vi "[Template] - State Machine Module.vi"() -> ()   [LabVIEW 2015]
uses:
  TypeDefs/ENUM_State Template.ctl
  TypeDefs/ENUM_Request Template.ctl
  Utility/Universal Utility/FP/FPClass/(FP)/DecFrame_FP/DecFrame_FP.lvclass
  <vilib>/Utility/error.llb/DialogType.ctl
  Utility/Universal Utility/TypeDefs_Utility/ENUM RB_Pos_Quadrant Position.ctl
  <vilib>/Utility/error.llb/Trim Whitespace.vi
panel:
  in  "stop":bool
  out "Version":string
  out "Action":string
  out "Next Request":T1 caption="Request ENUM (REPLACE)"
  out "State":T2=enum."Idle" caption="State ENUM (REPLACE)"
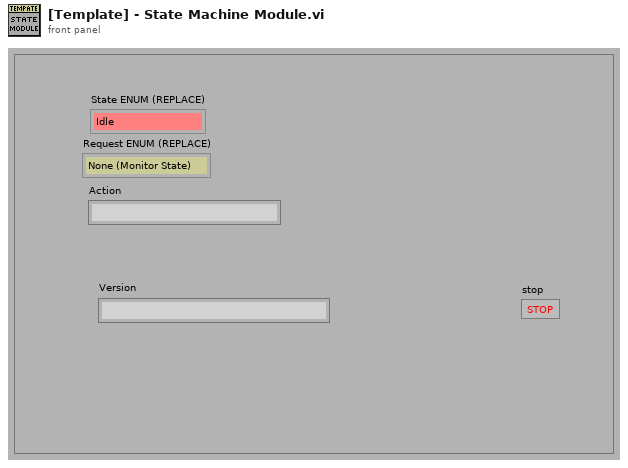
[diagram p1: front panel]
types:
  T1 = typedef "ENUM_Request Template.ctl" = enum16{"None (Monitor State)", "Request 1", "Stop Program", "SetFP Request"}
  T2 = typedef "ENUM_State Template.ctl" = enum16{"<Startup>", "Idle", "STATE 1", "<Shutdown>"}
  T3 = enum32{"invalid app kind", "Development System", "Run Time System", "Student Edition", "Embedded LabVIEW", "Evaluation", "Custom"}
  T4 = cluster{"App Kind":enum32{"invalid app kind", "Development System", "Run Time System", "Student Edition", "Embedded LabVIEW", "Evaluation", "Custom"}, "This VI":refnum<vi>, "Timeout":i32, "State":T2, "Request Q":refnum<queue>, "FP Data":refnum<class "DecFrame_FP.lvclass">}
  T5 = typedef "ENUM RB_Pos_Quadrant Position.ctl" = enum32{"LFT-TOP", "MID-TOP", "RGT-TOP", "LFT-CTR", "MID-CTR", "RGT-CTR", "LFT-BOT", "MID-BOT", "RGT-BOT"}
  T6 = enum32{"Invalid", "Standard", "Closed", "Hidden", "Minimized", "Maximized"}
  T7 = typedef "DialogType.ctl" = u16
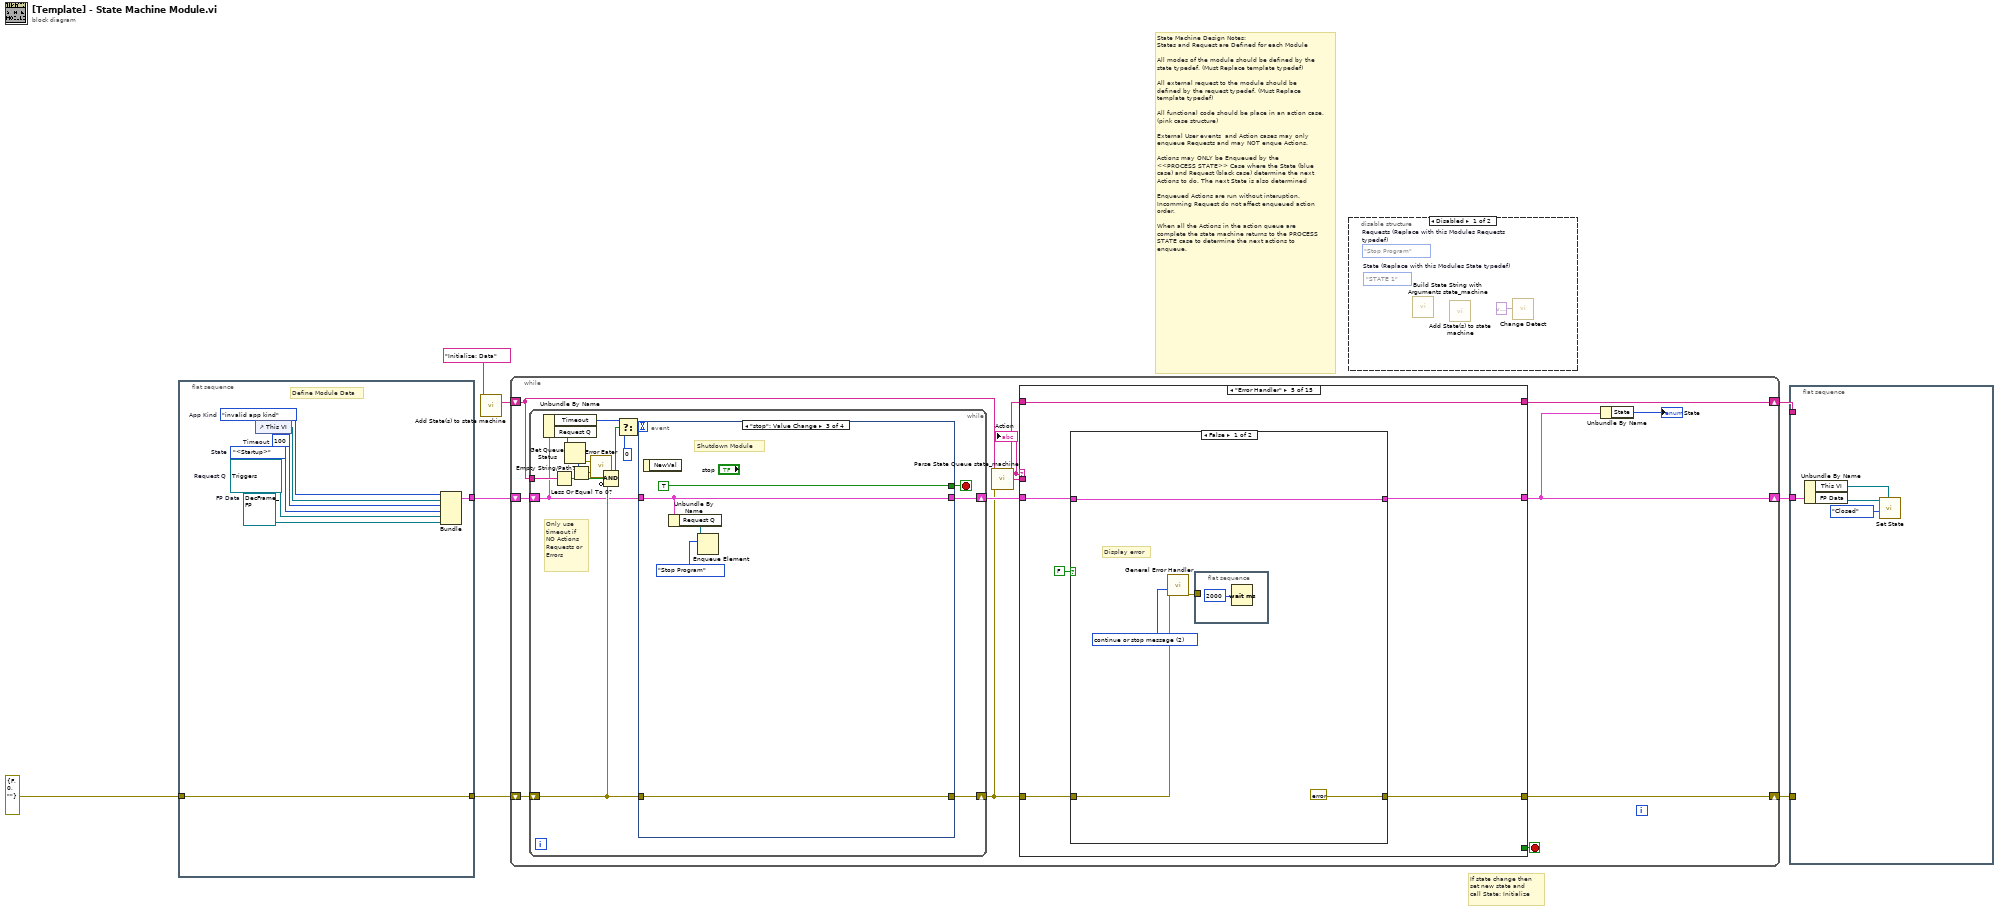
[diagram p0: block diagram]
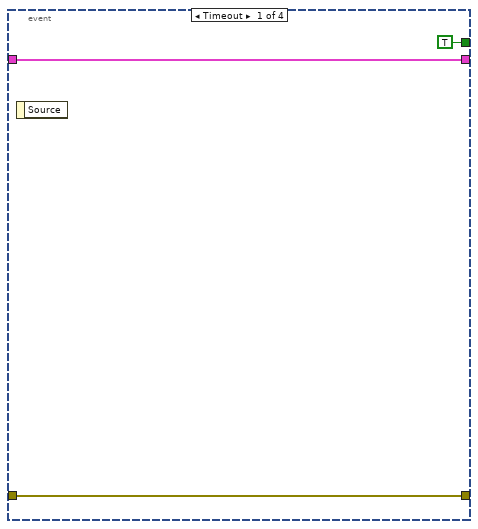
[diagram p3: hidden frame]
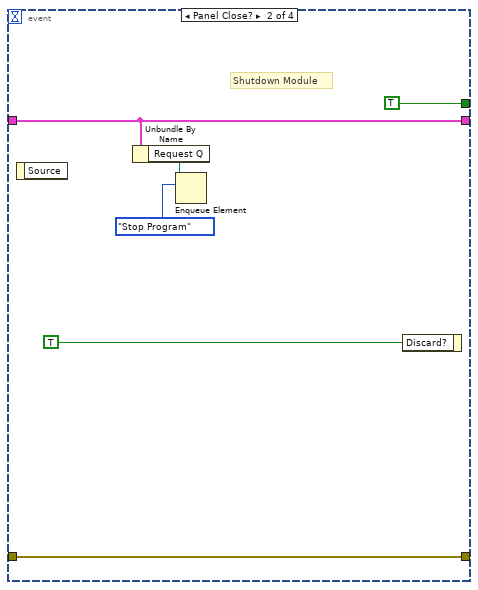
[diagram p4: hidden frame]
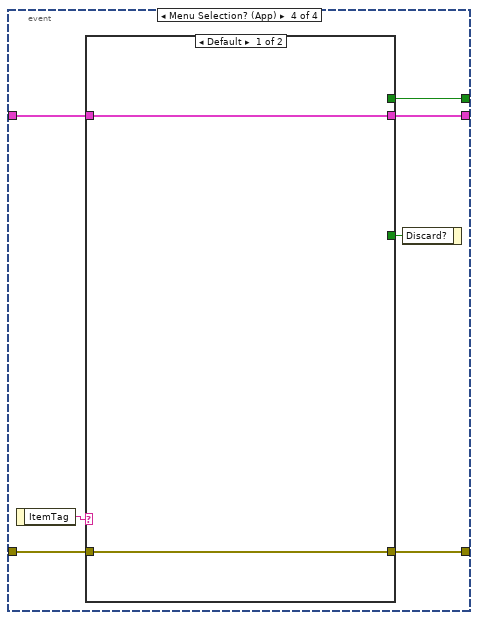
[diagram p5: hidden frame]
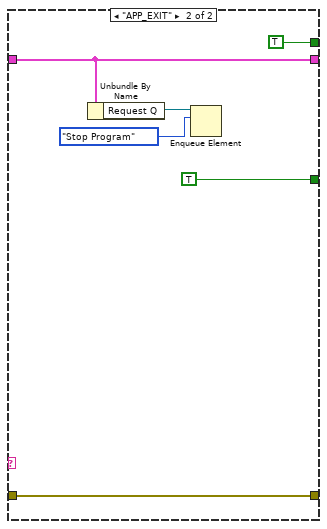
[diagram p6: hidden frame]
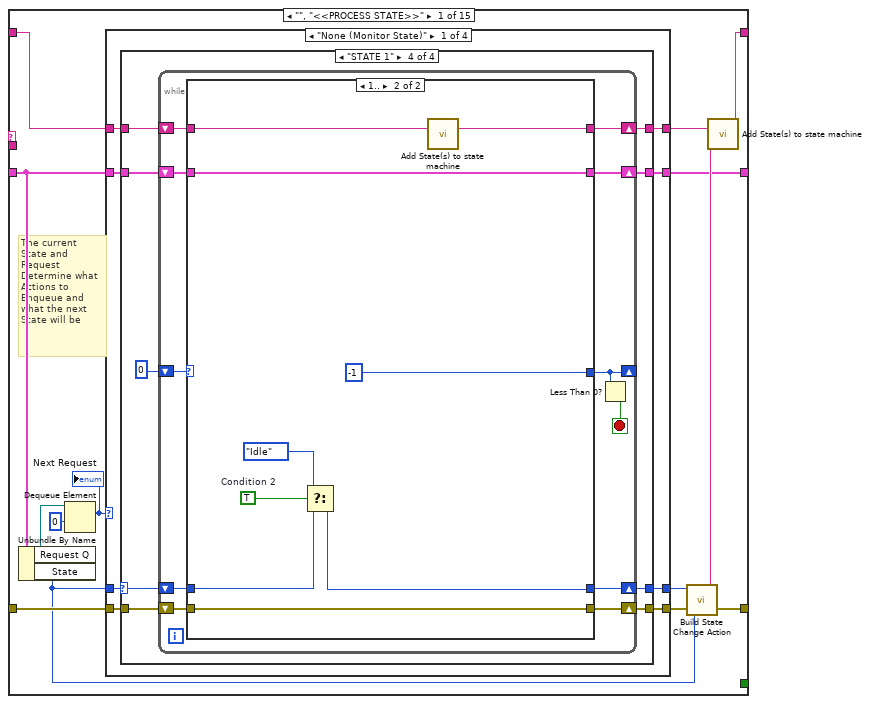
[diagram p7: hidden frame]
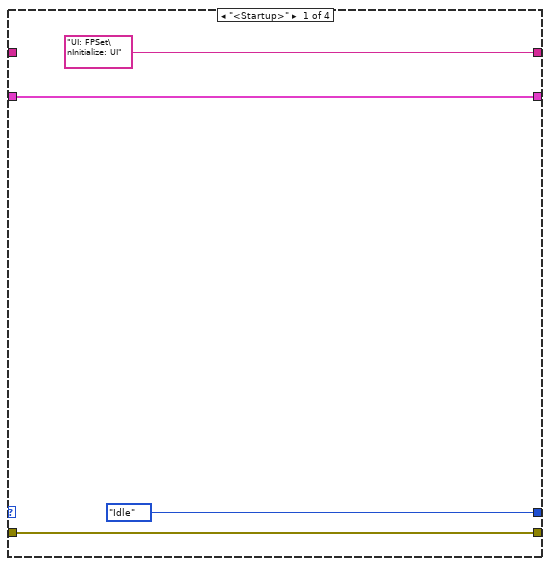
[diagram p8: hidden frame]
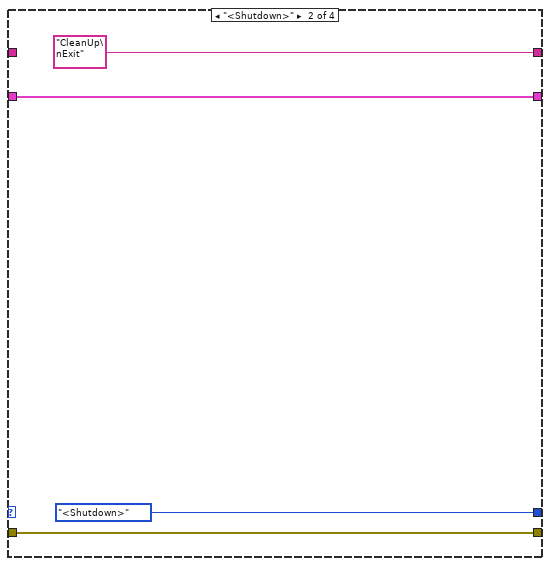
[diagram p9: hidden frame]
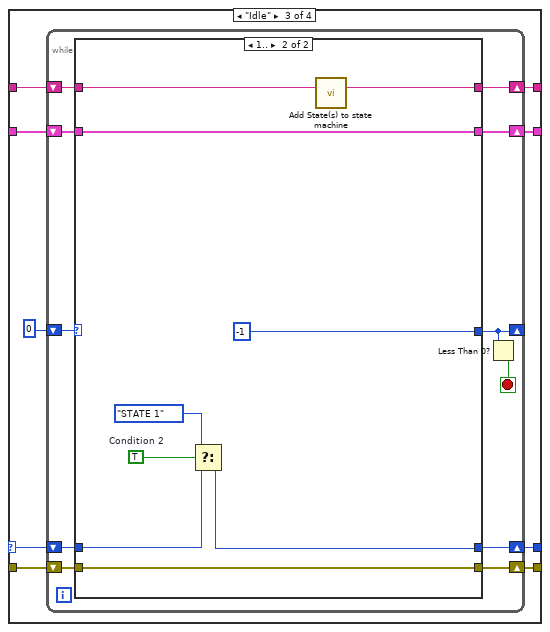
[diagram p10: hidden frame]
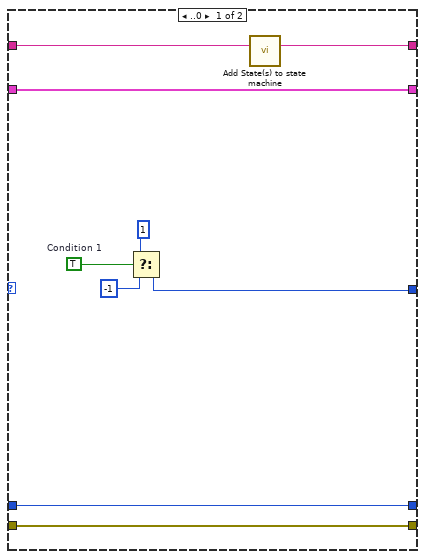
[diagram p11: hidden frame]
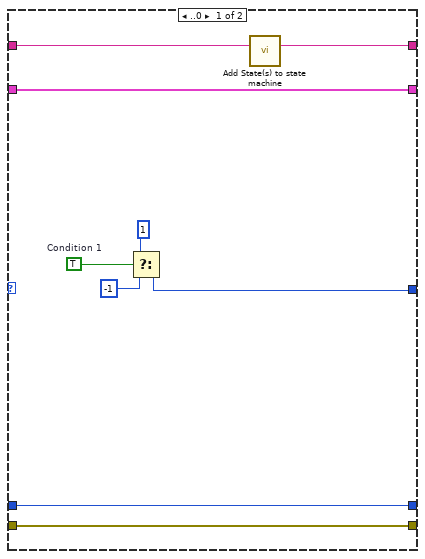
[diagram p12: hidden frame]
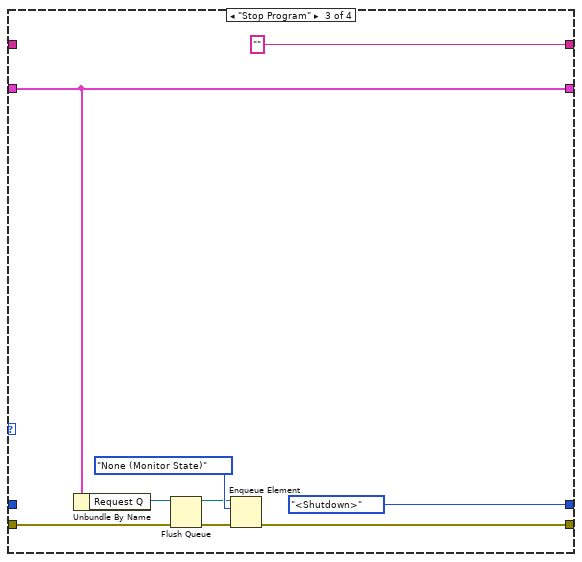
[diagram p17: hidden frame]
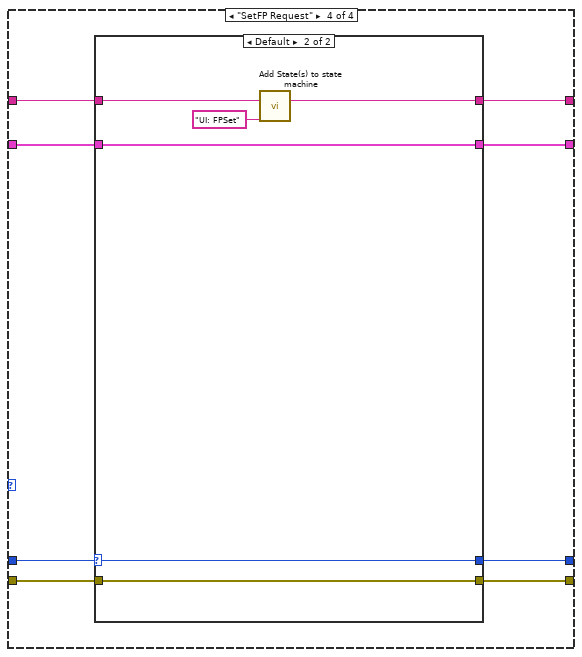
[diagram p18: hidden frame]
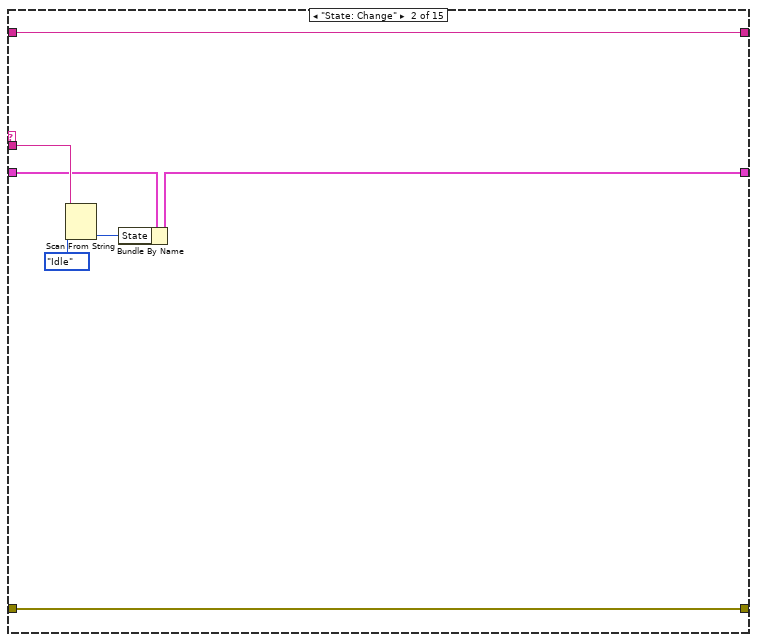
[diagram p20: hidden frame]
diagram:
  # "If state change then \nset new state and \ncall State: Initialize"
  # "State Machine Design Notes:\nStates and Request are Defined for each Module\n\nAll modes of the module should be defined by the state typedef. (Must Replace template typedef)\n\nAll external request to the module should be\ndefined by the request typedef. (Must Replace template typedef)\n\nAll functional code should be place in an action case. (pink case structure)\n\nExternal User events  and Action cases may only enqueue Requests and may NOT enque Actions.\n\nActions may ONLY be Enqueued by the\n<<PROCESS STATE>> Case where the State (blue case) and Request (black case) determine the next Actions to do. The next State is also determined\n\nEnqueued Actions are run without interuption.\nIncomming Request do not affect enqueued action order.\n\nWhen all the Actions in the action queue are complete the state machine returns to the PROCESS STATE case to determine the next actions to enqueue."
  n1 = flat-sequence {
    tunnel: errorcluster {"status"=FALSE, "code"=0, "source"=""} ("Error") -> [w16]
    tunnel: [w16] -> w6
    tunnel: [w15] -> w5
    frame #0 {
      w9 = refnum<class "DecFrame_FP.lvclass"> refnum  # FP Data
      w11 = refnum<queue> refnum items=["None (Monitor State)", "Request 1", "Stop Program", "SetFP Request"]  # Request Q
      w10 = ENUM_State_Template."<Startup>"  # State
      w13 = T3."invalid app kind"  # App Kind
      w14 = 100  # Timeout
      # "Define Module Data"
      n2 = control-ref of="This VI"() -> (w12:refnum<vi>)
      n3 = Bundle("App Kind"=w13, "This VI"=w12, "Timeout"=w14, "State"=w10, "Request Q"=w11, "FP Data"=w9) -> (w15:T4)  [unwired: 1 in]
    }
  }
  n4 = call "Add State(s) to state machine.vi"("State(s) in Front (\"\")"="Initialize: Data") -> ("States Out"=w8:string)  [unwired: 14 in]
  n5 = while "JKI - String-Based Queued State Machine (Basic) v1.0" {
    shift-right: [w17] -> w3
    shift-left: w5 -> [w25]
    shift-right: [w18] -> w2
    shift-left: w6 -> [w24]
    shift-right: [w27] -> w1
    shift-left: w8 -> [w20]
    stop <- w26 stop-if-true
    n6 = while {
      shift-right: [w43] -> w22
      shift-left: w24 -> [w36]
      shift-right: [w44] -> w23
      shift-left: w25 -> [w34]
      tunnel: w20 -> [w40]
      stop <- w37 stop-if-true
      # "Only use\ntimeout if\nNO Actions\nRequests or\nErrors"
      n7 = Unbundle By Name(w34) -> ("Timeout"=w38:i32, "Request Q"=w32:refnum<queue>)
      n8 = Empty String/Path?(string/path=w40) -> (empty?=w33:bool)
      n9 = Get Queue Status(queue=w32) -> (error out=w30:errorcluster, # elements in queue=w35:i32)  [unwired: 2 in, 6 out]
      n10 = Less Or Equal To 0?(x=w35) -> (x <= 0?=w31:bool)
      n11 = call "Error Eater.vi"("error in (no error)"=w30) -> ()  [unwired: 2 in]
      n12 = Compound Arithmetic op=AND(w31, w33, invert w36) -> (w42:bool)
      n13 = Select(t=w38, s=w42, f=0) -> (s? t:f=w39:i32)
      n14 = event shown="[2] \"stop\": Value Change" {
        selector: _ -> [_ _ _ _]
        dyn-events: _ -> [_ _ _ _]
        timeout: w39 -> [_ _ _ _]
        tunnel: w34 -> [w46 w51 w57 w62]
        tunnel: [w47 w53 w58 w64] -> w43
        tunnel: w36 -> [w47 w53 w58 w65]
        tunnel: [w46 w51 w57 w61] -> w44
        tunnel: [TRUE TRUE TRUE w59] -> w37
        event Timeout {
          n15 = event-data() -> ()  [unwired: 1 in, 1 out]
        }
        event Panel Close? {
          # "Shutdown Module"
          n16 = event-data() -> ()  [unwired: 1 in, 1 out]
          n17 = Unbundle By Name(w51) -> ("Request Q"=w49:refnum<queue>)
          n18 = Enqueue Element(queue=w49, element=ENUM_Request_Template."Stop Program") -> ()  [unwired: 2 in, 3 out]
          n19 = event-data("Discard?"=TRUE) -> ()  [unwired: 1 in, 1 out]
        }
        event "stop": Value Change {
          # "Shutdown Module"
          n20 = event-data() -> ()  [unwired: 1 in, 1 out]
          n21 = Unbundle By Name(w57) -> ("Request Q"=w55:refnum<queue>)
          n22 = Enqueue Element(queue=w55, element=ENUM_Request_Template."Stop Program") -> ()  [unwired: 2 in, 3 out]
        }
        event Menu Selection? (App) {
          n23 = event-data() -> ("ItemTag"=w63:string)  [unwired: 1 in]
          n24 = case shown="Default" w63 {
            tunnel: [w67 w73] -> w64
            tunnel: w65 -> [w67 w73]
            tunnel: [_ TRUE] -> w60
            tunnel: w62 -> [w66 w70]
            tunnel: [w66 w70] -> w61
            tunnel: [_ TRUE] -> w59
            frame Default {
            }
            frame "APP_EXIT" {
              n25 = Unbundle By Name(w70) -> ("Request Q"=w69:refnum<queue>)
              n26 = Enqueue Element(queue=w69, element=ENUM_Request_Template."Stop Program") -> ()  [unwired: 2 in, 3 out]
            }
          }
          n27 = event-data("Discard?"=w60) -> ()  [unwired: 1 in, 1 out]
        }
      }
    }
    n28 = call "Parse State Queue state_machine.vi"("State Queue"=w20, "Error In (no error)"=w22) -> ("Remaining States"=w29:string, "Current State"=w19:string, "Arguments"=w28:string)  [unwired: 11 in]
    "Action" <- w19
    n29 = case shown="\"Error Handler\"" w19 {
      selector: w19 -> [_ _ _ w258 _ _ _ _ _ _ _ _ _ _ _]
      tunnel: w29 -> [w77 w236 w239 w257 w267 w286 w288 w292 w306 w309 w312 w323 w324 w328 w331]
      tunnel: w28 -> [_ w235 _ _ _ _ _ _ _ _ _ _ _ _ _]
      tunnel: w23 -> [w78 w234 w243 w260 w270 w281 w291 w293 w303 w311 w313 w318 w325 w327 w330]
      tunnel: [w79 w237 w240 w262 w268 w285 w290 w294 w295 w310 w314 w319 w326 w329 w332] -> w18
      tunnel: w22 -> [w82 w237 w241 w261 w271 w285 w290 w294 w295 w310 w314 w320 w326 w329 w332]
      tunnel: [w86 w236 w238 w257 w267 w286 w288 w292 w306 w309 w312 w323 w324 w328 w331] -> w27
      tunnel: [_ _ _ _ _ _ TRUE _ _ _ _ _ _ _ _] -> w26
      tunnel: [w75 w233 w242 w260 w269 w281 w291 w293 w307 w311 w313 w317 w325 w327 w330] -> w17
      frame "", "<<PROCESS STATE>>" {
        # "The current\nState and \nRequest\nDetermine what\nActions to\nEnqueue and\nwhat the next\nState will be"
        n30 = Unbundle By Name(w78) -> ("Request Q"=w84:refnum<queue>, "State"=w81:T2)
        n31 = Dequeue Element(queue=w84, timeout in ms (-1)=0) -> (element=w74:T1)  [unwired: 1 in, 3 out]
        "Next Request" <- w74
        n32 = case shown="\"None (Monitor State)\"" w74 {
          selector: w74 -> [_ w180 _ _]
          tunnel: w77 -> [w91 w187 _ w217]
          tunnel: [w88 w186 w211 w216] -> w75
          tunnel: [w92 w185 w204 w213] -> w79
          tunnel: w82 -> [w93 w184 w205 w214]
          tunnel: w81 -> [w94 w183 _ w219]
          tunnel: [w87 w182 ENUM_State_Template."<Shutdown>" ("State") w215] -> w80
          tunnel: w78 -> [w89 w181 w211 w218]
          tunnel: [w90 w179 "" ("Remaining States") w220] -> w76
          frame "None (Monitor State)" {
            n33 = case shown="\"STATE 1\"" w94 {
              selector: w94 -> [_ _ w109 w147]
              tunnel: w93 -> [w98 w102 w108 w146]
              tunnel: [w98 w102 w104 w142] -> w92
              tunnel: w91 -> [_ _ w111 w149]
              tunnel: ["UI: FPSet\nInitialize: UI" "CleanUp\nExit" w106 w144] -> w90
              tunnel: w89 -> [w97 w101 w110 w148]
              tunnel: [w97 w101 w105 w143] -> w88
              tunnel: [ENUM_State_Template."Idle" ("State") ENUM_State_Template."<Shutdown>" ("State") w103 w141] -> w87
              frame "<Startup>" {
              }
              frame "<Shutdown>" {
              }
              frame "Idle" {
                n34 = while {
                  shift-right: [w114] -> w104
                  shift-left: w108 -> [w115]
                  shift-right: [w116] -> w103
                  shift-left: w109 -> [w117]
                  shift-right: [w112] -> w105
                  shift-left: w110 -> [w113]
                  shift-right: [w120] -> w106
                  shift-left: w111 -> [w121]
                  shift-right: [w118] -> _
                  shift-left: 0 -> [w122]
                  stop <- w119 stop-if-true
                  n35 = case shown="1.." w122 {
                    tunnel: w121 -> [w131 w140]
                    tunnel: [w130 w139] -> w120
                    tunnel: [w125 -1 ("t")] -> w118
                    tunnel: w117 -> [w123 w134]
                    tunnel: [w123 w133] -> w116
                    tunnel: w115 -> [w129 w138]
                    tunnel: [w129 w138] -> w114
                    tunnel: w113 -> [w128 w137]
                    tunnel: [w128 w137] -> w112
                    frame ..0 {
                      w124 = TRUE  # Condition 1
                      n36 = Select(t=1, s=w124, f=-1) -> (s? t:f=w125:i32)
                      n37 = call "Add State(s) to state machine.vi"("State(s) in (\"\")"=w131) -> ("States Out"=w130:string)  [unwired: 14 in]
                    }
                    frame 1.. {
                      w136 = TRUE  # Condition 2
                      n38 = Select(t=ENUM_State_Template."STATE 1", s=w136, f=w134) -> (s? t:f=w133:T2)
                      n39 = call "Add State(s) to state machine.vi"("State(s) in (\"\")"=w140) -> ("States Out"=w139:string)  [unwired: 14 in]
                    }
                  }
                  n40 = Less Than 0?(x=w118) -> (x < 0?=w119:bool)
                }
              }
              frame "STATE 1" {
                n41 = while {
                  shift-right: [w152] -> w142
                  shift-left: w146 -> [w153]
                  shift-right: [w154] -> w141
                  shift-left: w147 -> [w155]
                  shift-right: [w150] -> w143
                  shift-left: w148 -> [w151]
                  shift-right: [w158] -> w144
                  shift-left: w149 -> [w159]
                  shift-right: [w156] -> _
                  shift-left: 0 -> [w160]
                  stop <- w157 stop-if-true
                  n42 = case shown="1.." w160 {
                    tunnel: w159 -> [w169 w178]
                    tunnel: [w168 w177] -> w158
                    tunnel: [w163 -1 ("t")] -> w156
                    tunnel: w155 -> [w161 w172]
                    tunnel: [w161 w171] -> w154
                    tunnel: w153 -> [w167 w176]
                    tunnel: [w167 w176] -> w152
                    tunnel: w151 -> [w166 w175]
                    tunnel: [w166 w175] -> w150
                    frame ..0 {
                      w162 = TRUE  # Condition 1
                      n43 = Select(t=1, s=w162, f=-1) -> (s? t:f=w163:i32)
                      n44 = call "Add State(s) to state machine.vi"("State(s) in (\"\")"=w169) -> ("States Out"=w168:string)  [unwired: 14 in]
                    }
                    frame 1.. {
                      w174 = TRUE  # Condition 2
                      n45 = Select(t=ENUM_State_Template."Idle", s=w174, f=w172) -> (s? t:f=w171:T2)
                      n46 = call "Add State(s) to state machine.vi"("State(s) in (\"\")"=w178) -> ("States Out"=w177:string)  [unwired: 14 in]
                    }
                  }
                  n47 = Less Than 0?(x=w156) -> (x < 0?=w157:bool)
                }
              }
            }
          }
          frame "Request 1" {
            n48 = case shown="\"Idle\"" w183 {
              selector: w183 -> [w189 w192 w196 w200]
              tunnel: w187 -> [w191 w195 w198 w202]
              tunnel: w181 -> [w190 w194 w199 w203]
              tunnel: [w190 w194 w199 w203] -> w186
              tunnel: [w191 w195 w198 w202] -> w179
              tunnel: [w188 w193 w197 w201] -> w185
              tunnel: w184 -> [w188 w193 w197 w201]
              tunnel: w180 -> [_ _ _ _]
              tunnel: [w189 w192 w196 w200] -> w182
              frame "Idle" {
              }
              frame "STATE 1" {
              }
              frame "<Shutdown>" {
              }
              frame "<Startup>" {
              }
            }
          }
          frame "Stop Program" {
            n49 = Unbundle By Name(w211) -> ("Request Q"=w208:refnum<queue>)
            n50 = Flush Queue(queue=w208, error in (no error)=w205) -> (queue out=w207:refnum<queue>, error out=w206:errorcluster)  [unwired: 1 out]
            n51 = Enqueue Element(queue=w207, element=ENUM_Request_Template."None (Monitor State)", error in (no error)=w206) -> (error out=w204:errorcluster)  [unwired: 1 in, 2 out]
          }
          frame "SetFP Request" {
            n52 = case shown="Default" w219 {
              selector: w219 -> [w221 w226]
              tunnel: [w223 w229] -> w220
              tunnel: w218 -> [w222 w227]
              tunnel: w217 -> [w223 w230]
              tunnel: [w222 w227] -> w216
              tunnel: [w221 w226] -> w215
              tunnel: w214 -> [w224 w225]
              tunnel: [w224 w225] -> w213
              frame "<Shutdown>" {
              }
              frame Default {
                n53 = call "Add State(s) to state machine.vi"("State(s) in (\"\")"=w230, "State(s) at Back (\"\")"="UI: FPSet") -> ("States Out"=w229:string)  [unwired: 13 in]
              }
            }
          }
        }
        n54 = call "Build State Change Action.vi"("Current State"=w81, "Target State"=w80) -> ("Action String Out"=w85:string)  [unwired: 3 in]
        n55 = call "Add State(s) to state machine.vi"("State(s) in (\"\")"=w76, "State(s) at Back (\"\")"=w85) -> ("States Out"=w86:string)  [unwired: 13 in]
      }
      frame "State: Change" {
        n56 = Scan From String(input string=w235, default 1=ENUM_State_Template."Idle" ("State")) -> (output 1=w231:T2)  [unwired: 3 in, 3 out]
        n57 = Bundle By Name(cluster=w234, "State"=w231) -> (w233:T4)
      }
      frame "State: Initialize" {
        n58 = Unbundle By Name(w243) -> ("State"=w244:T2)
        n59 = case shown="\"<Shutdown>\"" w244 {
          tunnel: w243 -> [w247 w250 w253 w256]
          tunnel: [w247 w250 w253 w256] -> w242
          tunnel: w241 -> [w246 w249 w252 w255]
          tunnel: [w246 w249 w252 w255] -> w240
          tunnel: w239 -> [w245 w248 w251 w254]
          tunnel: [w245 w248 w251 w254] -> w238
          frame "Idle" {
          }
          frame "<Startup>" {
          }
          frame "STATE 1" {
          }
          frame "<Shutdown>" {
          }
        }
      }
      frame Default {
        w265 = 42 items=["No error", "Argument error", "Memory is full", "Out of zone", "End of file", "File already open", "Generic file I/O error", "File not found", "File permission error", "Disk is full", "Duplicate path", "Too many files open", "System feature not enabled", "Resource file not found", "Cannot add resource", "Resource not found", "Image not found", "Image memory error", "Pen does not exist", "Config type invalid", "Config token not found", "Config parse error", "Config memory error", "Bad external code format", "Bad external code offset", "External code not present", "Null window", "Destroy window error", "Null menu", "Print aborted", "Bad print record", "Print driver error", "Windows error during printing", "Memory error during printing", "Print dialog error", "Generic print error", "Invalid device refnum", "Device not found", "Device parameter error", "Device unit error", "Cannot open device", "Device call aborted", "Generic error", "Cancelled by user", "Object ID too low", "Object ID too high", "Object not in heap", "Unknown heap", "Unknown object (invalid DefProc)", "Unknown object (DefProc not in table)", "Message out of range", "Invalid (null) method", "Unknown message", "Manager call not supported", "Bad address", "Network operation in progress", "Network operation timed out", "Connection is busy", "Network attribute not supported", "Network error", "Address in use", "System out of memory", "Connection aborted", "Connection refused", "Not connected", "Already connected", "Connection closed", "Initialization error (interapplication manager)", "Bad occurrence", "Wait on unbound occurrence handler", "Occurrence queue overflow", "Datalog type conflict", "Unused", "Unrecognized type (interapplication manager)", "Memory corrupt", "Failed to make temporary DLL", "Old CIN version", "Drag socket not found", "Failed to load drop-object", "Failed to register OLE object", "Failed to release OLE object", "Format specifier type mismatch", "Unknown format specifier", "Too few format specifiers", "Too many format specifiers", "Scan failed", "Newer CIN version", "Error converting to variant", "Runtime menu error", "Password tampered", "Variant attribute not found", "Incompatible variant data type", "Event data is not available", "Event Store is not present", "Occurrence is not found", "Event Queue is not created", "Event info is not available", "Refnum passed is NULL", "Error retrieving Class GUID", "Error retrieving CoClass GUID", "Error retrieving TypeLib GUID.", "Bad built application magic bytes.", "Specific driver is different from the specific driver associated with the Logical Name.", "There is no session opened to the class driver.", "Max Error", "MAX - Error with config objects", "MAX - Error loading configuration", "MAX - Group not supported"]
        n60 = Format Into String(format string="Unable to process Action\nNo Action Case is defined for\n%s" ("message"), error in=w261, w258) -> (resulting string=w264:string, error out=w263:errorcluster)  [unwired: 1 in]
        n61 = call <vilib>:"Error Cluster From Error Code.vi"("show call chain? (False)"=TRUE, "error in (no error)"=w263, "error message (\"\")"=w264, "error code (0)"=w265) -> ("error out"=w262:errorcluster)  [unwired: 5 in]
      }
      frame "Error Handler" {
        n62 = case shown="False" FALSE {
          tunnel: w271 -> [w277 _]
          tunnel: [w276 w279] -> w269
          tunnel: w270 -> [w276 w279]
          tunnel: [errorcluster {"status"=FALSE, "code"=0, "source"=""} ("error out") errorcluster {"status"=FALSE, "code"=0, "source"=""} ("error out")] -> w268
          frame False {
            w273 = T7 2 items=["no dialog", "OK message", "continue or stop message", "OK message + warnings", "continue/stop + warnings"] ("type of dialog (OK msg:1)")
            # "Display error"
            n63 = call <vilib>:"General Error Handler.vi"("type of dialog (OK msg:1)"=w273, "error in (no error)"=w277) -> ("error out"=w274:errorcluster)  [unwired: 9 in, 4 out]
            n64 = flat-sequence {
              tunnel: w274 -> [_]
              frame #0 {
                n65 = Wait (ms)(milliseconds to wait=u32 2000) -> ()  [unwired: 1 out]
              }
            }
          }
          frame True {
            # "Clear error"
          }
        }
      }
      frame "CleanUp" {
        # "Destroy and open refs"
        n66 = Unbundle By Name(w281) -> ("This VI"=w287:refnum<vi>, "Request Q"=w283:refnum<queue>)
        n67 = Close Reference(reference=w287) -> (error out=w284:errorcluster)  [unwired: 1 in]
        n68 = Release Queue(queue=w283) -> (error out=w282:errorcluster)  [unwired: 2 in, 2 out]
        n69 = call <vilib>:"Clear Errors.vi"("error in (no error)"=w284) -> ()  [unwired: 5 in, 2 out]
        n70 = call <vilib>:"Clear Errors.vi"("error in (no error)"=w282) -> ()  [unwired: 5 in, 2 out]
      }
      frame "Exit" {
      }
      frame "---------- Initialize ----------" {
      }
      frame "Initialize: Data" {
        w296 = i16 -2  # Border Spacing
        w300 = 0  # Decoration Index
        w301 = u16 0  # Monitor #
        # "INI Data"
        n71 = Unbundle By Name(w303) -> ("FP Data"=w302:refnum<class "DecFrame_FP.lvclass">)
        n72 = call-dynamic "Setup DecFrame Data.vi"("Border Spacing"=w296, "Monitor #"=w301, "FPLocation"=ENUM_RB_Pos_Quadrant_Position."LFT-TOP", "Decoration Index"=w300, "(FP)"=w302) -> ("(FP) Out"=w298:refnum<class "DecFrame_FP.lvclass">)  [unwired: 5 in, 1 out]
        n73 = property class="App"() -> ("App.Kind"=w299:T3)  [unwired: 2 in, 2 out]
        n74 = Obtain Queue(element data type=ENUM_Request_Template."Request 1" ("Triggers")) -> (queue out=w305:refnum<queue>)  [unwired: 4 in, 2 out]
        n75 = Bundle By Name(cluster=w303, "FP Data"=w298, "App Kind"=w299, "Request Q"=w305) -> (w307:T4)
      }
      frame "Initialize: UI" {
        # "Setup UI indicators and controls"
        n76 = call "[Version] - Get Application Main.vi"() -> ("Version"=→"Version":string)
      }
      frame "---------- UI ----------" {
      }
      frame "UI: FPSet" {
        # "Set FP"
        n77 = Unbundle By Name(w318) -> ("This VI"=w322:refnum<vi>, "FP Data"=w321:refnum<class "DecFrame_FP.lvclass">)
        n78 = call-dynamic "Set State.vi"("VI Ref"=w322, "Error"=w320, "State"=T6."Standard", "(FP)"=w321) -> ("Error Out"=w319:errorcluster, "(FP) Out"=w316:refnum<class "DecFrame_FP.lvclass">)  [unwired: 5 in, 1 out]
        n79 = Bundle By Name(cluster=w318, "FP Data"=w316) -> (w317:T4)
      }
      frame "---------- Action ----------" {
      }
      frame "Action: One" {
      }
      frame "Action: Two" {
      }
    }
    n80 = Unbundle By Name(w17) -> ("State"=→"State":T2)
  }
  n81 = disable-structure shown="Disabled" {
    frame Disabled {
      (unwired) ENUM_Request_Template."Stop Program"  # Requests (Replace with this Modules Requests typedef)
      (unwired) ENUM_State_Template."STATE 1"  # State (Replace with this Modules State typedef)
      n82 = call "Build State String with Arguments state_machine.vi"() -> ()  [unwired: 6 in, 1 out]
      n83 = call "Add State(s) to state machine.vi"() -> ()  [unwired: 15 in, 1 out]
      n84 = call "Change Detect.vi"("Value"=variant) -> ()  [unwired: 4 in, 1 out]
    }
    frame Enabled {
    }
  }
  n85 = flat-sequence {
    tunnel: w3 -> [w337]
    tunnel: w2 -> [_]
    tunnel: w1 -> [_]
    frame #0 {
      n86 = Unbundle By Name(w337) -> ("This VI"=w335:refnum<vi>, "FP Data"=w336:refnum<class "DecFrame_FP.lvclass">)
      n87 = call-dynamic "Set State.vi"("VI Ref"=w335, "State"=T6."Closed", "(FP)"=w336) -> ()  [unwired: 6 in, 3 out]
    }
  }
